vi "Savitsky Golay Weighted Filter (single).vi"(4 "Window Order":i32, 6 "Side Points Unit (points)":enum16{"Points", "Data"}(ring), 8 "error in (no error)":errorcluster, 9 "polynomial order (3)":i32=3, 10 "side points (6)":dbl=6.0, 11 "XY-data":cluster{"X-array":dbl[], "Y-array":dbl[]}) -> (0 "error out":errorcluster, 3 "XY-data out":cluster{"X-array":dbl[], "Y-array":dbl[]} {"Y-array" format="%.2p"; "X-array" format="%.2p"})   [LabVIEW 2019, in "xy_utilities.lvlib"]
doc: "Filter <b>XY-data</b>'s Y-Array with a Savitsky-Golay FIR smoothing filter.\n\n<b>side points</b> specifies the number of data points to each side of the current data point to use for the least squares minimization. side points*2 + 1 is the length of the moving window, which must be greater than the polynomial order.\n\n<b>polynomial order</b> specifies the order of the polynomial. \n\nWire data to the data input to determine the polymorphic instance to use or manually select the instance."
uses:
  xy_utilities.lvlib
  <vilib>/Analysis/NI_AALBase.lvlib
  <vilib>/Analysis/3filter.llb/Savitzky-Golay Filter (DBL).vi
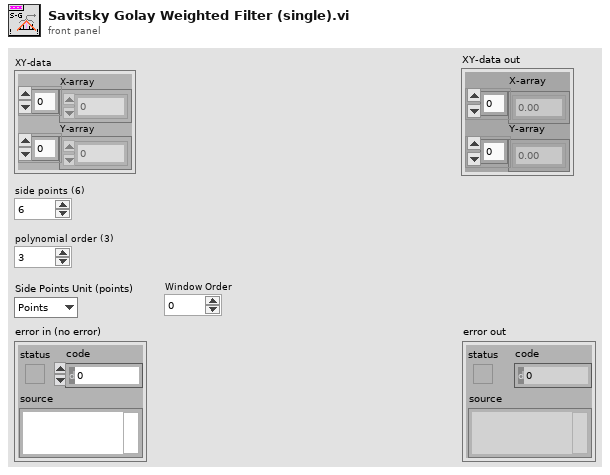
[diagram p1: front panel]
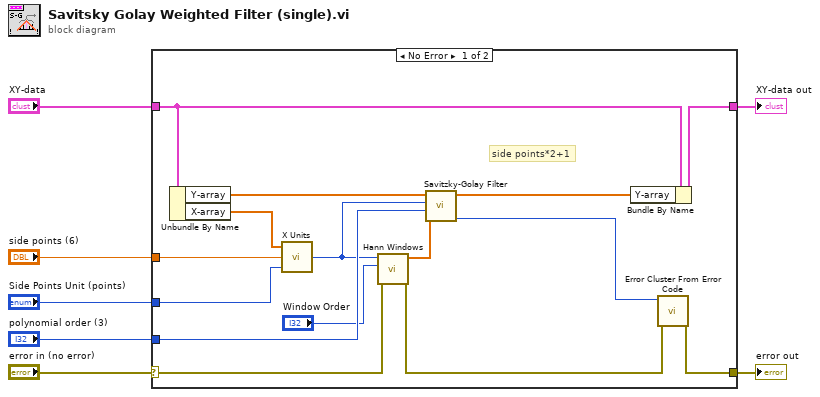
[diagram p0: block diagram]
diagram:
  n1 = case shown="No Error" "error in (no error)" {
    selector: "error in (no error)" -> [w10 w24]
    tunnel: [w17 w24] -> w6
    tunnel: "XY-data" -> [w21 w23]
    tunnel: [w22 w23] -> w4
    tunnel: "side points (6)" -> [w15 _]
    tunnel: "Side Points Unit (points)" -> [w14 _]
    tunnel: "polynomial order (3)" -> [w13 _]
    frame No Error {
      # "side points*2+1"
      n2 = Unbundle By Name(w21) -> ("Y-array"=w20:dbl[], "X-array"=w16:dbl[])
      n3 = call "X Units.vi"("Interval Units (points)"=w14, "Interval (h)"=w15, "X-array"=w16) -> ("h (points)"=w12:i32)
      n4 = call "Hann Windows.vi"("error in (no error)"=w10, "Window Order"="Window Order", "side points (6)"=w12) -> ("error out"=w9:errorcluster, "Window"=w11:dbl[])  [unwired: 7 in]
      n5 = call-poly <vilib>:"Savitzky-Golay Filter.vi"("Weight"=w11, "polynomial order"=w13, "side points"=w12, "X"=w20) -> ("error"=w18:i32, "Filtered X"=w19:dbl[])  [unwired: 6 in]
      n6 = Bundle By Name(cluster=w21, "Y-array"=w19) -> (w22:cluster{"X-array":dbl[], "Y-array":dbl[]})
      n7 = call <vilib>:"Error Cluster From Error Code.vi"("error in (no error)"=w9, "error code (0)"=w18) -> ("error out"=w17:errorcluster)  [unwired: 7 in]
    }
    frame Error {
    }
  }
  "error out" <- w6
  "XY-data out" <- w4
